vi "ErorLogger.vi"(11 "error in (no error)":errorcluster) -> ()   [LabVIEW 2024]
uses:
  <vilib>/Utility/error.llb/DialogType.ctl
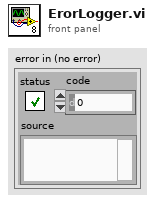
[diagram p1: front panel]
types:
  T1 = typedef "DialogType.ctl" = u16
  T2 = enum16{"open", "replace", "create", "open or create", "replace or create", "replace or create with confirmation"}
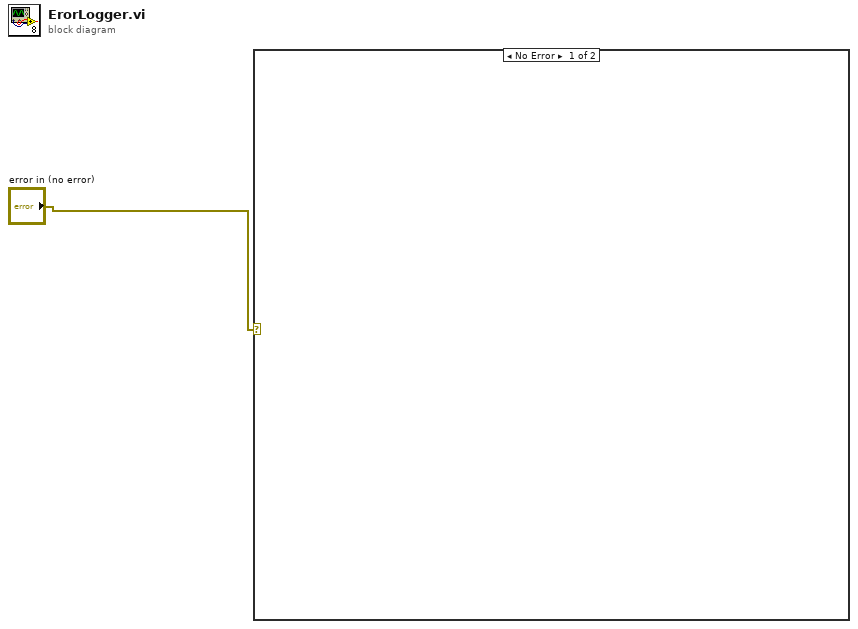
[diagram p0: block diagram]
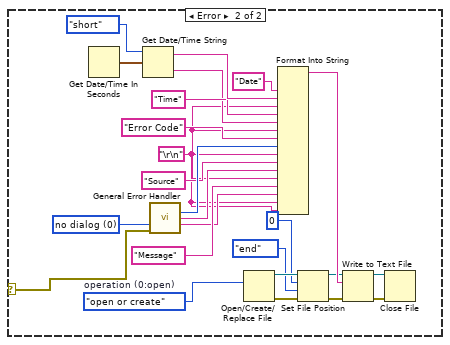
[diagram p2: hidden frame]
diagram:
  n1 = case shown="No Error" "error in (no error)" {
    selector: "error in (no error)" -> [_ w3]
    frame No Error {
    }
    frame Error {
      w4 = T1 0 items=["no dialog", "OK message", "continue or stop message", "OK message + warnings", "continue/stop + warnings"] ("type of dialog (OK msg:1)")
      w2 = "\r\n"
      w26 = T2."open or create"  # operation (0:open)
      n2 = Get Date/Time In Seconds() -> (seconds since 1Jan1904=w23:timestamp)
      n3 = Get Date/Time String(date format (0)=enum16{"short", "long", "abbreviated"}."short", seconds (now)=w23) -> (date string=w20:string, time string=w18:string)  [unwired: 1 in]
      n4 = call <vilib>:"General Error Handler.vi"("type of dialog (OK msg:1)"=w4, "error in (no error)"=w3) -> ("code out"=w16:i32, "source out"=w14:string, "message"=w12:string)  [unwired: 9 in, 2 out]
      n5 = Open/Create/Replace File(operation (0:open)=w26) -> (refnum out=w10:refnum<file>, error out=w9:errorcluster)  [unwired: 5 in, 1 out]
      n6 = Format Into String("Date" ("input 1"), w20, w2, "Time" ("input 3"), w18, w2, "Error Code", w16, w2, "Source" ("input 10"), w14, w2, "Message" ("input 13"), w12, w2, w2) -> (resulting string=w11:string)  [unwired: 3 in, 1 out]
      n7 = Set File Position(offset (in bytes) (0)=i64 0, refnum=w10, from (0:start)=enum16{"start", "end", "current"}."end", error in=w9) -> (refnum out=w7:refnum<file>, error out=w8:errorcluster)
      n8 = Write to Text File(file (use dialog)=w7, text=w11, error in=w8) -> (refnum out=w25:refnum<file>, error out=w24:errorcluster)  [unwired: 1 in, 1 out]
      n9 = Close File(refnum=w25, error in=w24) -> ()  [unwired: 2 out]
    }
  }
